vi "Create Device.vi"(8 "error in (no error)":errorcluster, 10 "DevInfo":refnum<class "DevInfo.lvclass">, 11 "Controller in":refnum<class "Controller.lvclass">) -> (0 "error out":errorcluster, 1 "created?":bool, 2 "Device Obj":refnum<class "Hardware.lvclass">, 3 "Controller out":refnum<class "Controller.lvclass">)   [LabVIEW 2016, in "Controller Actor.lvlib" / "Controller.lvclass"]
uses:
  <userlib>/Common Components/Controller/Controller.lvclass
  <userlib>/Common Components/Hardware/DevInfo/DevInfo.lvclass
  <userlib>/Common Components/Hardware/Abstract Hardware/Hardware.lvclass
  <userlib>/Common Components/Hardware/DevInfo/DevInfo.lvclass/DevInfo.ctl
  <userlib>/Common Components/Hardware/DevInfo/Read Device Name.vi
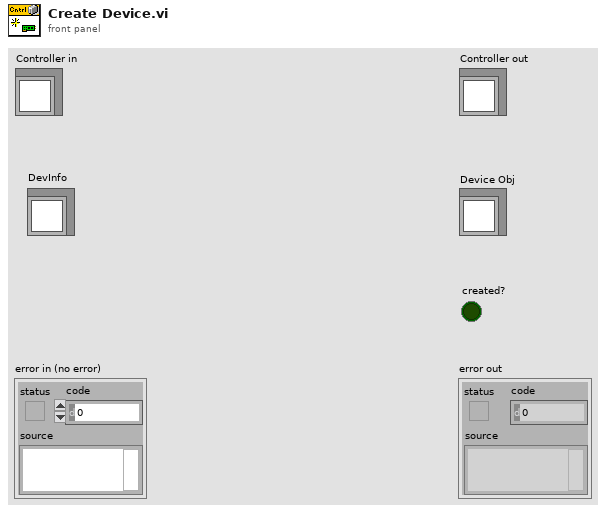
[diagram p1: front panel]
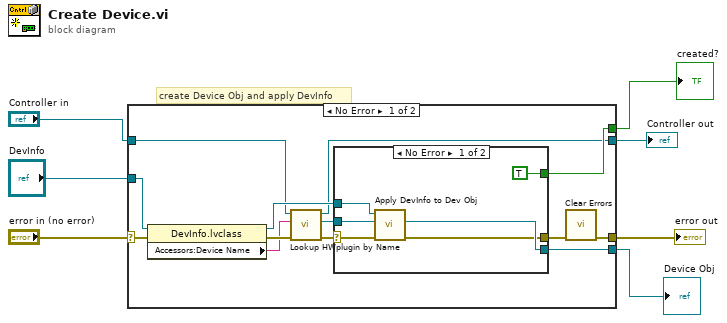
[diagram p0: block diagram]
diagram:
  # "create Device Obj and apply DevInfo"
  n1 = case shown="No Error" "error in (no error)" {
    selector: "error in (no error)" -> [w15 w29]
    tunnel: [w16 w29] -> w2
    tunnel: [w8 w28] -> w5
    tunnel: "Controller in" -> [w9 w28]
    tunnel: "DevInfo" -> [w20 _]
    tunnel: [w19 _] -> w3
    tunnel: [w17 _] -> w1
    frame No Error {
      n2 = property class="DevInfo.lvclass"(reference=w20, error in=w15) -> (reference out=w10:refnum<class "DevInfo.lvclass">, error out=w14:errorcluster, "Accessors:Device Name"=w11:string)
      n3 = call <userlib>:"Lookup HWplugin by Name.vi"("error in (no error)"=w14, "Device Name"=w11, "Controller in"=w9) -> ("error out"=w13:errorcluster, "Hardware.lvclass"=w12:refnum<class "Hardware.lvclass">, "Controller out"=w8:refnum<class "Controller.lvclass">)  [unwired: 6 in]
      n4 = case shown="No Error" w13 {
        selector: w13 -> [w22 w27]
        tunnel: w12 -> [w24 _]
        tunnel: [w23 _] -> w19
        tunnel: [w21 w27] -> w18
        tunnel: [TRUE _] -> w17
        tunnel: w10 -> [w25 _]
        frame No Error {
          n5 = call <userlib>:"Apply DevInfo to Dev Obj.vi"("error in (no error)"=w22, "Dev Obj in"=w24, "DevInfo in"=w25) -> ("error out"=w21:errorcluster, "Dev Obj out"=w23:refnum<class "Hardware.lvclass">)  [unwired: 6 in, 1 out]
        }
        frame Error {
        }
      }
      n6 = call <vilib>:"Clear Errors.vi"("error in (no error)"=w18) -> ("error out"=w16:errorcluster)  [unwired: 5 in, 1 out]
    }
    frame Error {
    }
  }
  "error out" <- w2
  "Controller out" <- w5
  "Device Obj" <- w3
  "created?" <- w1
